vi "10.vi"() -> ()   [LabVIEW 2021]
uses:
  <vilib>/gmath/NI_AAL_MathFunc.lvlib
panel:
  out "Numeric":u64
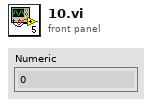
[diagram p1: front panel]
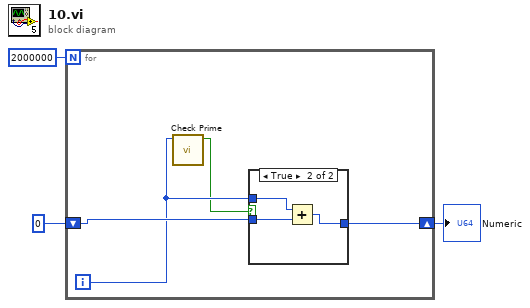
[diagram p0: block diagram]
diagram:
  n1 = for {
    N: 2000000 -> [_]
    shift-right: [w5] -> w1
    shift-left: u64 0 -> [w7]
    i -> [w6]
    n2 = call <vilib>:"Check Prime.vi"("n"=w6) -> ("prime?"=w4:bool)  [unwired: 10 in]
    n3 = case shown="True" w4 {
      tunnel: w7 -> [w8 w11]
      tunnel: w6 -> [_ w10]
      tunnel: [w8 w9] -> w5
      frame False {
      }
      frame True {
        n4 = Add(x=w10, y=w11) -> (x+y=w9:u64)
      }
    }
  }
  "Numeric" <- w1
